vi "read_params.vi"(8 "error in (no error)":errorcluster, 11 "KNeighborsClassifier in":refnum<class "KNeighborsClassifier.lvclass">) -> (0 "error out":errorcluster, 2 "params":T1={"n_neighbors"=5.0, "weights"="uniform", "algorithm"="auto", "leaf_size"=30.0, "p"=2.0, "metric"="minkowski", "n_jobs"=0.0}, 3 "KNeighborsClassifier out":refnum<class "KNeighborsClassifier.lvclass">)   [LabVIEW 2020, in "KNeighborsClassifier.lvclass"]
uses:
  KNeighborsClassifier.lvclass
  Controls/kneighbors_classifier_params.ctl
  KNeighborsClassifier.lvclass/KNeighborsClassifier.ctl
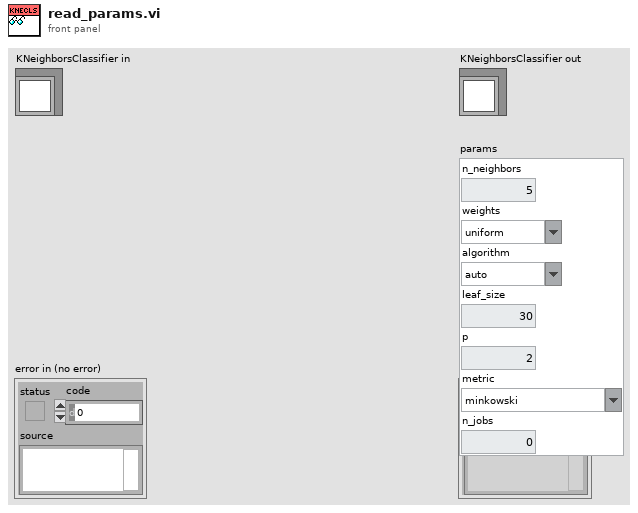
[diagram p1: front panel]
types:
  T1 = typedef "kneighbors_classifier_params.ctl" = cluster{"n_neighbors":dbl, "weights":string, "algorithm":string, "leaf_size":dbl, "p":dbl, "metric":string, "n_jobs":dbl}
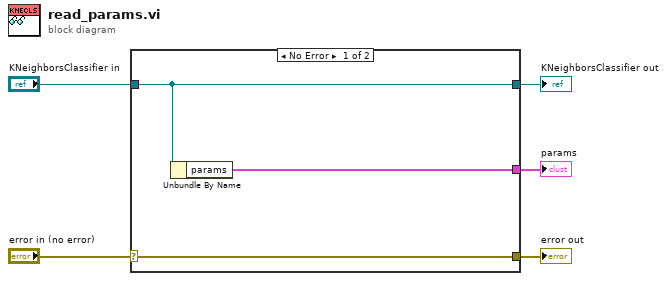
[diagram p0: block diagram]
diagram:
  n1 = case shown="No Error" "error in (no error)" {
    selector: "error in (no error)" -> [w8 w9]
    tunnel: [w8 w9] -> w4
    tunnel: [w7 w10] -> w2
    tunnel: "KNeighborsClassifier in" -> [w7 w10]
    tunnel: [w6 _] -> w1
    frame No Error {
      n2 = Unbundle By Name(w7) -> ("params"=w6:T1)
    }
    frame Error {
    }
  }
  "error out" <- w4
  "KNeighborsClassifier out" <- w2
  "params" <- w1
